vi "WatchMovie.vi"(8 "error in (no error)":errorcluster, 11 "Facade in":refnum<class "Facade.lvclass">) -> (0 "error out":errorcluster, 2 "ProcessMessage":string, 3 "Facade out":refnum<class "Facade.lvclass">)   [LabVIEW 2013, in "Facade.lvclass"]
uses:
  Facade.lvclass
  Facade.lvclass/Facade.ctl
  CDPlayer.lvclass/CDPlayer.lvclass
  Tuner.lvclass/Tuner.lvclass
  DVDPlayer.lvclass/DVDPlayer.lvclass
  Amplifer.lvclass/Amplifer.lvclass
  Projector.lvclass/Projector.lvclass
  RoomLight.lvclass/RoomLight.lvclass
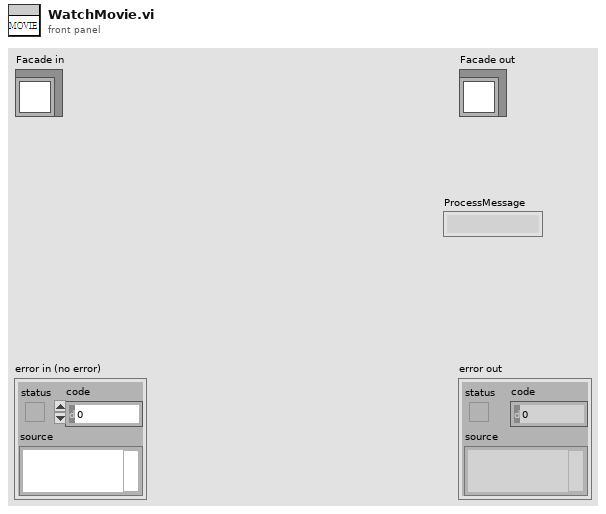
[diagram p1: front panel]
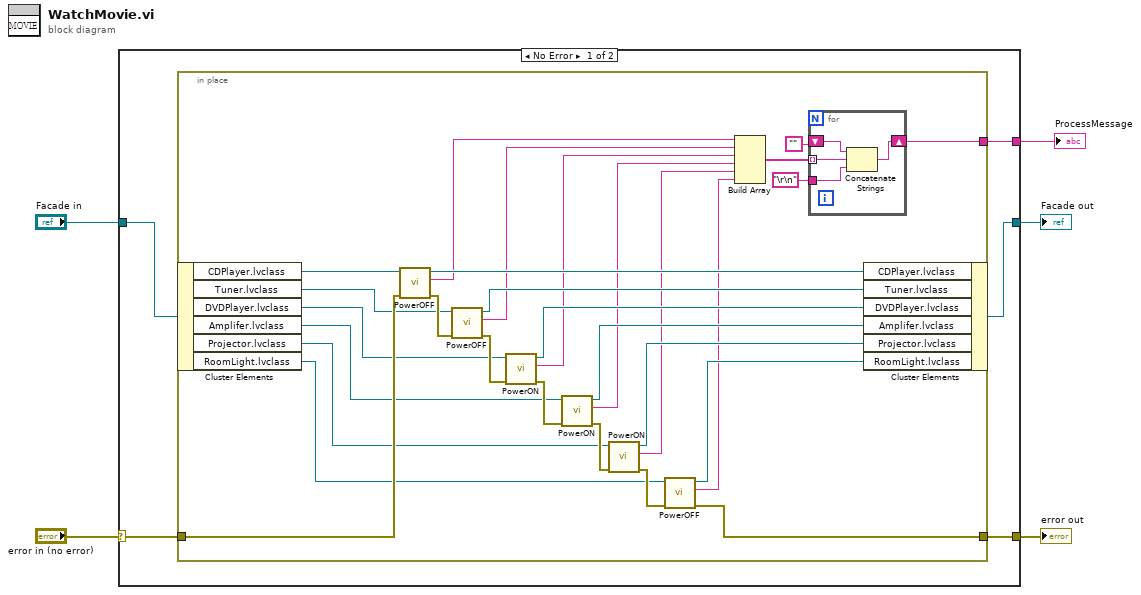
[diagram p0: block diagram]
diagram:
  n1 = case shown="No Error" "error in (no error)" {
    selector: "error in (no error)" -> [w10 w45]
    tunnel: [w8 w45] -> w4
    tunnel: [w7 w44] -> w2
    tunnel: "Facade in" -> [w9 w44]
    tunnel: [w6 _] -> w1
    frame No Error {
      n2 = in-place {
        in-place-border: w10 -> [w39]
        in-place-border: [w21] -> w8
        in-place-border: [w11] -> w6
        n3 = in-place-cluster #1(w9) -> ("CDPlayer.lvclass"=w33:refnum<class "CDPlayer.lvclass">, "Tuner.lvclass"=w32:refnum<class "Tuner.lvclass">, "DVDPlayer.lvclass"=w31:refnum<class "DVDPlayer.lvclass">, "Amplifer.lvclass"=w30:refnum<class "Amplifer.lvclass">, "Projector.lvclass"=w29:refnum<class "Projector.lvclass">, "RoomLight.lvclass"=w28:refnum<class "RoomLight.lvclass">)
        n4 = call-dynamic "PowerOFF.vi"("error in (no error)"=w39, "CDPlayer in"=w33) -> ("error out"=w38:errorcluster, "Message"=w20:string, "CDPlayer out"=w27:refnum<class "CDPlayer.lvclass">)  [unwired: 7 in]
        n5 = call-dynamic "PowerOFF.vi"("error in (no error)"=w38, "Tuner in"=w32) -> ("error out"=w37:errorcluster, "Message"=w19:string, "Tuner out"=w26:refnum<class "Tuner.lvclass">)  [unwired: 7 in]
        n6 = call-dynamic "PowerON.vi"("error in (no error)"=w37, "DVDPlayer in"=w31) -> ("error out"=w36:errorcluster, "Message"=w18:string, "DVDPlayer out"=w25:refnum<class "DVDPlayer.lvclass">)  [unwired: 7 in]
        n7 = call-dynamic "PowerON.vi"("error in (no error)"=w36, "Amplifer in"=w30) -> ("error out"=w35:errorcluster, "Message"=w17:string, "Amplifer out"=w24:refnum<class "Amplifer.lvclass">)  [unwired: 7 in]
        n8 = call-dynamic "PowerON.vi"("error in (no error)"=w35, "Projector in"=w29) -> ("error out"=w34:errorcluster, "Message"=w16:string, "Projector out"=w23:refnum<class "Projector.lvclass">)  [unwired: 7 in]
        n9 = call-dynamic "PowerOFF.vi"("error in (no error)"=w34, "RoomLight in"=w28) -> ("error out"=w21:errorcluster, "Message"=w15:string, "RoomLight out"=w22:refnum<class "RoomLight.lvclass">)  [unwired: 7 in]
        n10 = Build Array(w20, w19, w18, w17, w16, w15) -> (w14:string[])
        n11 = for {
          tunnel: w14 -> [w43] mode=indexing
          tunnel: "\r\n" -> [w42]
          shift-right: [w40] -> w11
          shift-left: "" -> [w41]
          n12 = Concatenate Strings(w41, w43, w42) -> (w40:string)
        }
        n13 = in-place-cluster #1("CDPlayer.lvclass"=w27, "Tuner.lvclass"=w26, "DVDPlayer.lvclass"=w25, "Amplifer.lvclass"=w24, "Projector.lvclass"=w23, "RoomLight.lvclass"=w22) -> (w7:refnum<class "Facade.lvclass">)
      }
    }
    frame Error {
    }
  }
  "error out" <- w4
  "Facade out" <- w2
  "ProcessMessage" <- w1
